vi "chirp_v0.vi"() -> ()   [LabVIEW 2014]
uses:
  <vilib>/rvi/FXPMathLib/FxpSinAndCos/XNode/nifxpmath_SinAndCos.xnode
  <vilib>/eio/EIONode/EIONode.xnode
  <vilib>/rvi/FXPMathLib/FxpMul/XNode/nifxpmath_Multiplier.xnode
  <vilib>/rvi/FXPMathLib/FxpSinAndCos/simVIs/DllFxpSinAndCosTemp_sub.vi
  <vilib>/rvi/FXPMathLib/FxpSinAndCos/subVIs/nifxpmath_SinAndCos_SimConfig.ctl
  <vilib>/rvi/eio/common/nirviEmuTemplateMethod_errors.vi
  <vilib>/rvi/FXPMathLib/sim/FxpSim.dll
  <vilib>/rvi/DataTransferAndStorage/Container/XNode/niFpgaContainer.xnode
  <vilib>/rvi/FXPMathLib/FxpSub/XNode/nifxpmath_Sub.xnode
  <vilib>/rvi/FXPMathLib/FxpAdd/XNode/nifxpmath_Add.xnode
  <vilib>/rvi/Analysis/measure/butterworth/XNode/niFpgaButterworthFilter.xnode
  <vilib>/rvi/interface/RandomDataEmulation/nirviRandomDataFpgaMultiElementTemplate.vi
panel:
  in  "Step/Chirp":bool
  in  "fb_step (N)":fxp<+/-,36,11>
  in  "initial frenqueny (Hz)":fxp<+,20,5>
  in  "target frenqueny (Hz)":fxp<+,23,8>
  in  "target time (s)":fxp<+,24,9>
  out "chirp_signal":fxp<+/-,36,11>
  out "frequency (Hz)":fxp<+,24,9>
  out "Load cell 1":fxp<+/-,60,14>
  out "Load cell 0":fxp<+/-,60,14>
  in  "xb_M_avg_Tc (uSec)":u32
  out "Omega_b(T)":fxp<+/-,20,9>
  out "Omega_b(M_avg)":fxp<+/-,32,12>
  out "Omega_b(M)":fxp<+/-,32,12>
  in  "Method case 2":i32
  out "f_LC":fxp<+/-,36,17>
  in  "Load cell reset":bool
  in  "Load cell stop":bool
  in  "Load cell start":bool
  out "fbr_d":fxp<+/-,36,13>
  in  "Sin wave amplitude (N)":fxp<+,20,11>
  out "Db_d(M_avg method)":fxp<+/-,25,10>
  in  "Db_d_M_Tc (mSec)":u32 format="%#_6f"
  out "Db_d(M method)":fxp<+/-,25,10>
  out "xb_d(M_avg method)":fxp<+/-,25,10>
  in  "Db_M_avg_Tc (uSec)":u32
  out "xb_d(M method)":fxp<+/-,25,10>
  in  "xb_d_M_Tc (mSec)":u32 format="%#_6f"
  in  "Method case":i32
  out "xb_d(T method)":fxp<+/-,25,10>
  out "Db_d(T method)":fxp<+/-,25,10>
  in  "mt0_velocity":u32
  out "mt_velocity":u32
  in  "mt0_omega":u32
  out "mt_omega":u32
  out "fbt_d":fxp<+/-,25,15>
  out "Db_d(mm/s)":fxp<+/-,25,10>
  out "Atom_Position_b":i32
  out "xb_d(mm/s)":fxp<+/-,25,10>
  in  "dF_PID_add":bool
  in  "scaled coefficients_dFb_PID":i32[](array[numeric])=[1067016412, 3362706]
  out "dFb_PID":fxp<+/-,25,15>
  out "Sin wave time (s)":fxp<+,64,32>
  in  "Atom Reset_b":bool
  out "xb(mm)":fxp<+/-,22,7>
  in  "Friction tolerance_b":fxp<+,12,4>
  in  "Coe Ini":bool
  in  "Encoder Reset_b":bool
  in  "Stop Motor_b":bool
  in  "viscous_cons_b":fxp<+/-,20,10>
  in  "fstb":fxp<+/-,15,6>
  in  "Db_d_tol":fxp<+,20,12>
  in  "Kib":fxp<+,27,10>
  in  "Kdb":fxp<+,26,2>
  in  "kb c":fxp<+,15,8>
  in  "kb t":fxp<+,15,8>
  out "fbt_i":fxp<+/-,34,18>
  in  "Kpb":fxp<+,11,7>=0.375
  in  "fv_coeff. b":fxp<+,13,1>
  out "Friction comp_b":fxp<+/-,20,10>
  in  "fcb":fxp<+/-,15,6>
  in  "fvb":fxp<+,20,12>
  out "kb":fxp<+,15,8>
  out "fb":fxp<+/-,20,10>
  out "fb_tilde":fxp<+/-,21,11>
  out "Fb_PID":fxp<+/-,21,11>
  in  "fb_tolerance":fxp<+,32,9>=1.0
  out "fbr":fxp<+/-,36,11>
  out "Encoder Position_b":i32
  out "rad(NrTheta)_b":fxp<+/-,33,18> format="%.21g"
  out "Db(mm)":fxp<+/-,22,7>
  out "Omega_b(rad/s)":fxp<+/-,20,9>
  out "vq_b_F":fxp<+/-,20,5> format="%.57g"
  out "vd_b_F":fxp<+/-,20,5>
  out "va_b":fxp<+/-,20,5> format="%.21g"
  out "vb_b":fxp<+/-,20,5> format="%.21g"
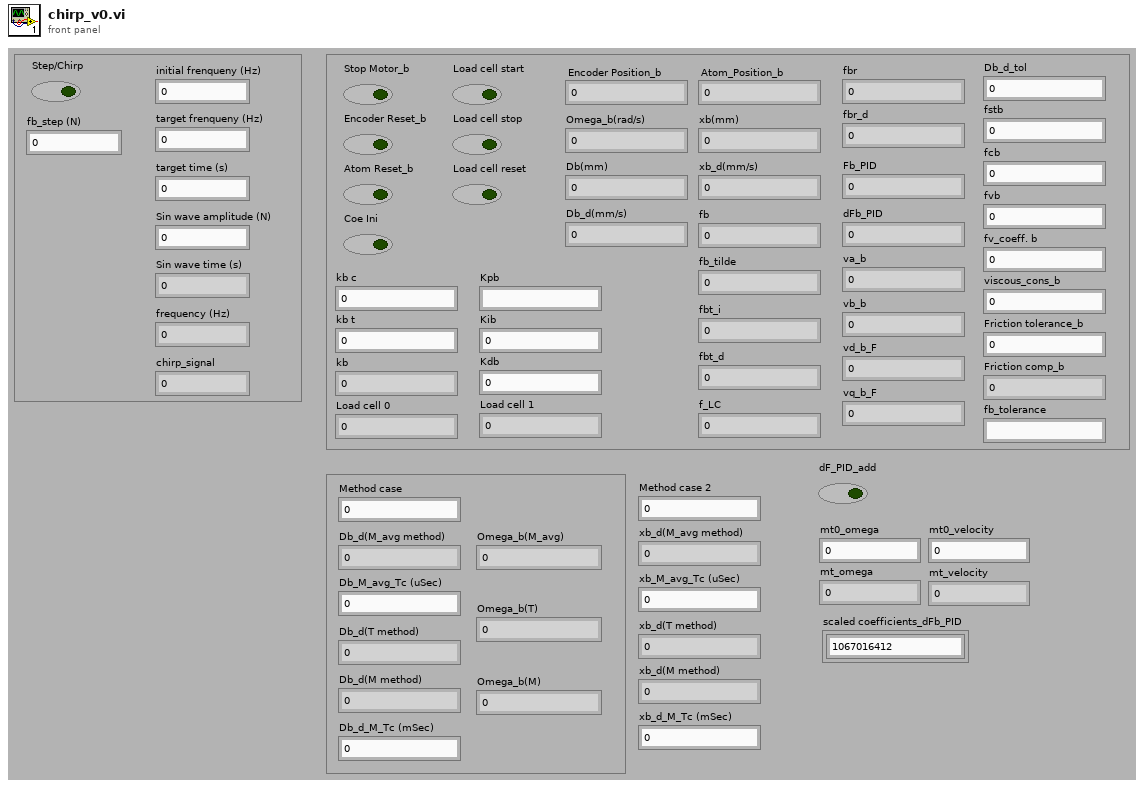
[diagram p1: front panel]
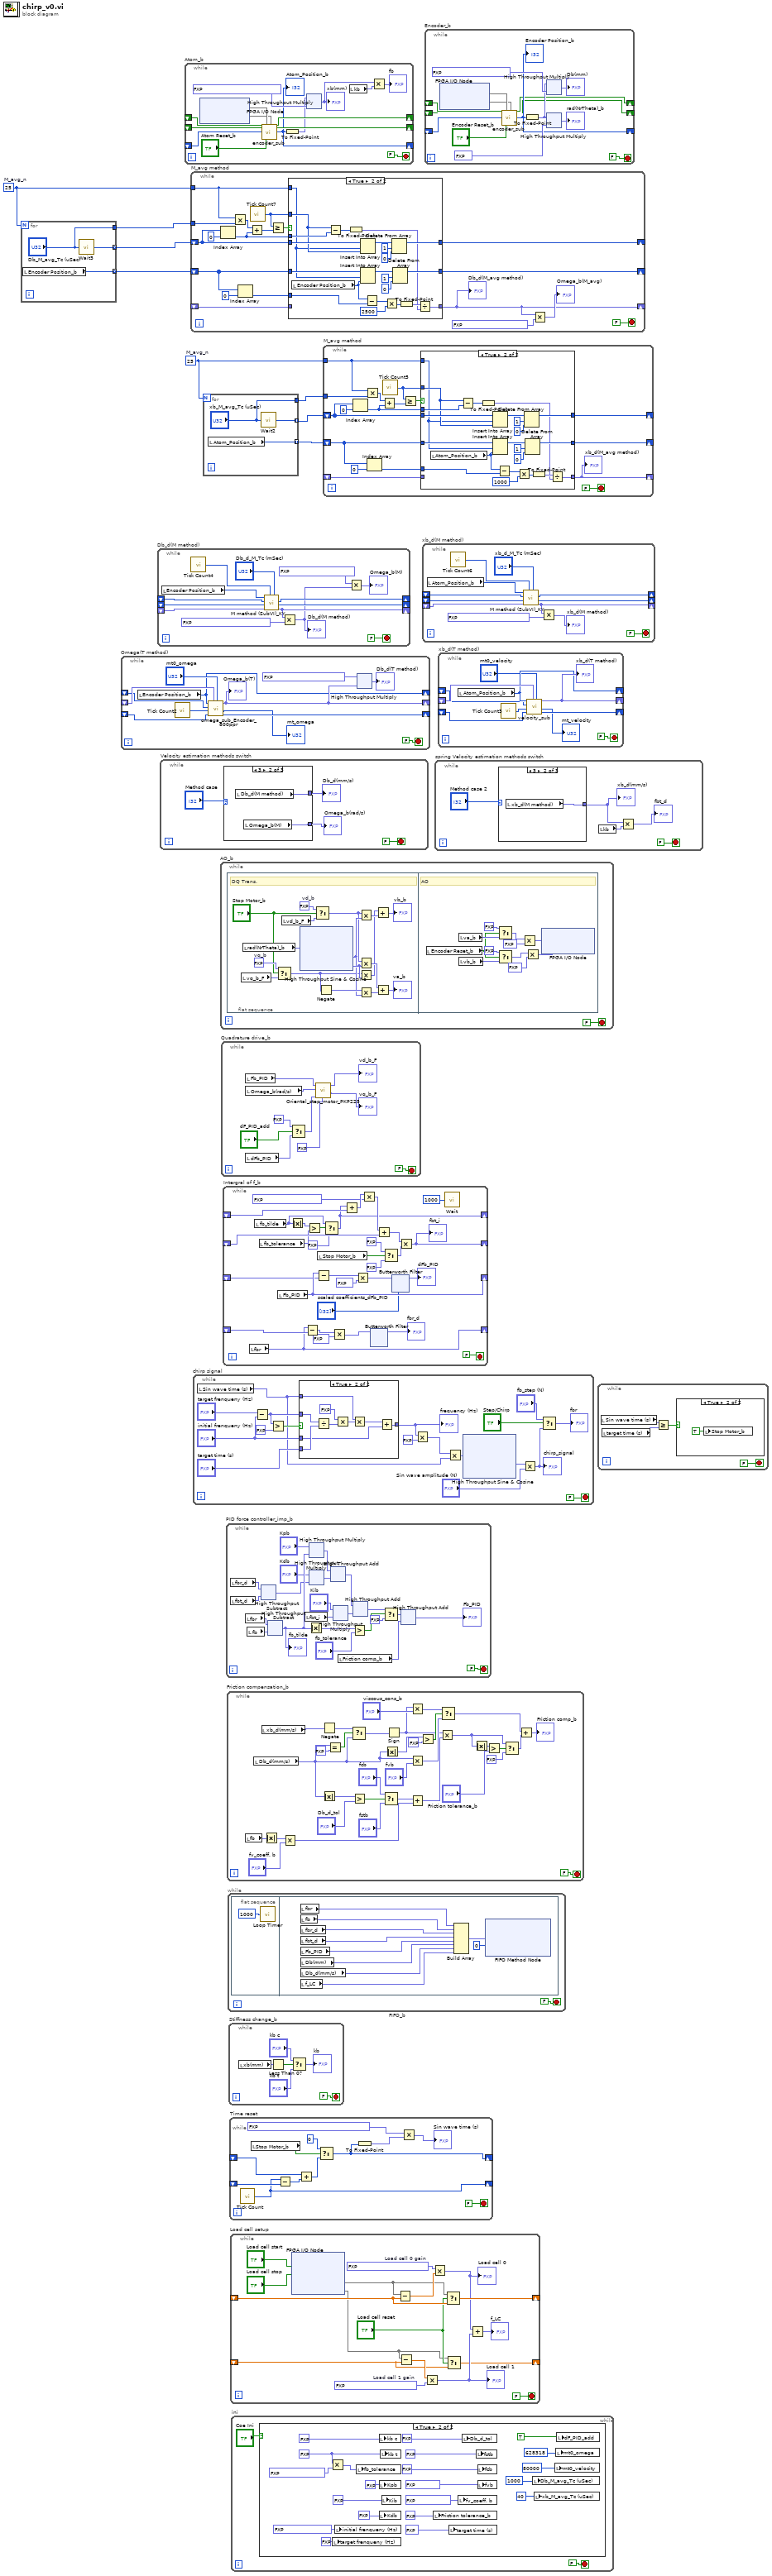
[diagram p0: block diagram]
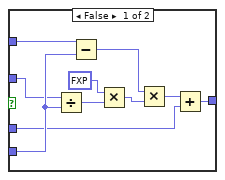
[diagram p3: hidden frame]
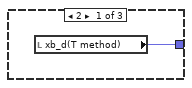
[diagram p5: hidden frame]
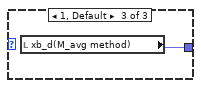
[diagram p6: hidden frame]
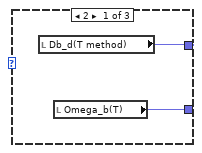
[diagram p8: hidden frame]
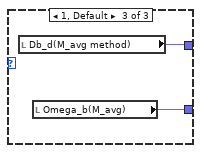
[diagram p9: hidden frame]
diagram:
  w2 = 25  # M_avg_n
  w6 = 25  # M_avg_n
  n1 = for {
    N: w6 -> [_]
    tunnel: [w11] -> w8 mode=indexing
    tunnel: [w9] -> w7 mode=indexing
    tunnel: ["Db_M_avg_Tc (uSec)"] -> w5
    n2 = local read "Encoder Position_b"() -> (w9:i32)
    n3 = call "Wait3"("Count(uSec)"="Db_M_avg_Tc (uSec)") -> ("Tick Count(uSec)"=w11:u32)
  }
  n4 = while "Omega(T method)" {
    shift-right: [w13] -> _
    shift-left: _ -> [w12]
    shift-right: [w20] -> _
    shift-left: _ -> [w14]
    shift-right: [w18] -> _
    shift-left: _ -> [w16]
    stop <- FALSE stop-if-true
    n5 = local read "Encoder Position_b"() -> (w13:i32)
    n6 = call "Tick Count2"() -> ("Tick Count(Ticks)"=w15:u32)
    n7 = call "omega_sub_Encoder_800ppr.vi"("mt0"="mt0_omega", "omega_pre"=w16, "ticks_m_pre"=w14, "ticks"=w15, "count_pre"=w12, "count"=w13) -> ("ticks_m"=w20:u32, "mt"=→"mt_omega":u32, "omega"=w18:fxp<+/-,20,9>)  [unwired: 3 in]
    "Omega_b(T)" <- w18
    n8 = xnode ("High Throughput Multiply")("x"=fxp<+/-,26,1> 0.38515496253967285, "y"=w18) -> ("x*y"=→"Db_d(T method)":fxp<+/-,24,9>)
  }
  n9 = while "Db_d(M method)" {
    shift-right: [w35] -> _
    shift-left: _ -> [w30]
    shift-right: [w34] -> _
    shift-left: _ -> [w29]
    shift-right: [w27] -> _
    shift-left: _ -> [w28]
    stop <- FALSE stop-if-true
    n10 = local read "Encoder Position_b"() -> (w31:i32)
    n11 = call "Tick Count4"() -> ("Tick Count(mSec)"=w32:u32)
    n12 = call "M method (SubVI)_KY.vi"("Tc (mSec)"="Db_d_M_Tc (mSec)", "Tick Count (mSec)"=w32, "Encoder velocity_pre (pulse/s)"=w28, "Shift Register in 2"=w29, "Shift Register in 1"=w30, "Encoder pulses"=w31) -> ("Encoder velocity (pulse/s)"=w27:fxp<+/-,64,32>, "Shift Register out 2"=w34:i32, "Shift Register out 1"=w35:u32)  [unwired: 3 in]
    n13 = Multiply(x=w27, y=fxp<+/-,20,-5> 0.002499997615814209) -> (x*y=w26:fxp<+/-,25,10>)
    "Db_d(M method)" <- w26
    n14 = Multiply(x=fxp<+/-,32,12> 3.1415929794311523, y=w26) -> (x*y=→"Omega_b(M)":fxp<+/-,32,12>)
  }
  n15 = while "Velocity estimation methods switch" {
    stop <- FALSE stop-if-true
    n16 = case shown="3" "Method case" {
      tunnel: [w42 w44 w46] -> w39
      tunnel: [w43 w45 w47] -> w38
      frame 2 {
        n17 = local read "Db_d(T method)"() -> (w42:fxp<+/-,25,10>)
        n18 = local read "Omega_b(T)"() -> (w43:fxp<+/-,20,9>)
      }
      frame 3 {
        n19 = local read "Db_d(M method)"() -> (w44:fxp<+/-,25,10>)
        n20 = local read "Omega_b(M)"() -> (w45:fxp<+/-,32,12>)
      }
      frame 1, Default {
        n21 = local read "Db_d(M_avg method)"() -> (w46:fxp<+/-,25,10>)
        n22 = local read "Omega_b(M_avg)"() -> (w47:fxp<+/-,32,12>)
      }
    }
    "Db_d(mm/s)" <- w39
    "Omega_b(rad/s)" <- w38
  }
  n23 = while "Atom_b" {
    shift-right: [w61] -> _
    shift-left: _ -> [w59]
    shift-right: [w60] -> _
    shift-left: _ -> [w58]
    shift-right: [w48] -> _
    shift-left: _ -> [w55]
    stop <- FALSE stop-if-true
    n24 = xnode "FPGA I/O Node"() -> ("Mod5/DI0"=w57, "Mod5/DI1"=w56)  [unwired: 2 in, 2 out]
    n25 = call "encoder_sub.vi"("A_pre"=w59, "B_pre"=w58, "Encoder Position_pre"=w55, "A input"=w57, "Encoder Position Reset"="Atom Reset_b", "B input"=w56) -> ("A"=w61:bool, "B"=w60:bool, "Encoder Position (Counts)"=w48:i32)  [unwired: 19 in]
    "Atom_Position_b" <- w48
    n26 = To Fixed-Point(number=w48) -> (fixed-point=w53:fxp<+/-,18,18>)  [unwired: 1 in]
    n27 = xnode ("High Throughput Multiply")("x"=w53, "y"=fxp<+/-,20,-5> 0.0009999871253967285) -> ("x*y"=w50:fxp<+/-,22,7>)
    "xb(mm)" <- w50
    n28 = local read "kb"() -> (w51:fxp<+,15,8>)
    n29 = Multiply(x=w50, y=w51) -> (x*y=→"fb":fxp<+/-,20,10>)
  }
  n30 = while "M_avg method" {
    shift-right: [w73] -> _
    shift-left: w8 -> [w76]
    tunnel: w6 -> [w74]
    shift-right: [w71] -> _
    shift-left: w7 -> [w69]
    shift-right: [w63] -> _
    shift-left: _ -> [w67]
    tunnel: w5 -> [w66]
    stop <- FALSE stop-if-true
    n31 = Index Array(array=w76, index=0) -> (element=w72:u32)
    n32 = Multiply(x=w74, y=w66) -> (x*y=w79:u32)
    n33 = Index Array(array=w69, index=0) -> (element=w68:i32)
    n34 = Add(x=w79, y=w72) -> (x+y=w78:u32)
    n35 = call "Tick Count7"() -> ("Tick Count(uSec)"=w75:u32)
    n36 = Greater Or Equal?(x=w75, y=w78) -> (x >= y?=w77:bool)
    n37 = case shown="True" w77 {
      tunnel: w76 -> [w84 w106]
      tunnel: w75 -> [_ w100]
      tunnel: w74 -> [_ w89]
      tunnel: [w84 w102] -> w73
      tunnel: w72 -> [_ w101]
      tunnel: w69 -> [w83 w90]
      tunnel: [w83 w88] -> w71
      tunnel: [w82 w87] -> w63
      tunnel: w68 -> [_ w85]
      tunnel: w67 -> [w82 _]
      frame False {
      }
      frame True {
        n38 = local read "Encoder Position_b"() -> (w94:i32)
        n39 = Subtract(x=w100, y=w101) -> (x-y=w99:u32)
        n40 = To Fixed-Point(number=w99) -> (fixed-point=w86:fxp<+,32,32>)  [unwired: 1 in]
        n41 = Insert Into Array(array=w106, index=w89, new element=w100) -> (w105:u32[])
        n42 = Insert Into Array(array=w90, index=w89, new element=w94) -> (w91:i32[])
        n43 = Subtract(x=w94, y=w85) -> (x-y=w95:i32)
        n44 = Multiply(x=w95, y=2500) -> (x*y=w97:i32)
        n45 = Delete From Array(array=w105, length=1, index=0) -> (array with subset deleted=w102:u32[])  [unwired: 1 out]
        n46 = Delete From Array(array=w91, length=1, index=0) -> (array with subset deleted=w88:i32[])  [unwired: 1 out]
        n47 = To Fixed-Point(number=w97) -> (fixed-point=w98:fxp<+/-,32,32>)  [unwired: 1 in]
        n48 = Divide(x=w98, y=w86) -> (x/y=w87:fxp<+/-,25,10>)
      }
    }
    "Db_d(M_avg method)" <- w63
    n49 = Multiply(x=w63, y=fxp<+/-,32,12> 3.1415929794311523 ("x")) -> (x*y=→"Omega_b(M_avg)":fxp<+/-,32,12>)
  }
  n50 = while "chirp signal" {
    stop <- FALSE stop-if-true
    n51 = local read "Sin wave time (s)"() -> (w107:fxp<+,64,32>)
    n52 = Subtract(x="target frenqueny (Hz)", y="initial frenqueny (Hz)") -> (x-y=w108:fxp<+/-,24,9>)
    n53 = Greater?(x=w108, y=fxp<+/-,24,9> 0.0) -> (0:w111:bool)
    n54 = case shown="True" w111 {
      tunnel: [w133 w142] -> w116
      tunnel: "target time (s)" -> [w130 w141]
      tunnel: "initial frenqueny (Hz)" -> [w129 w140]
      tunnel: w107 -> [w132 w139]
      tunnel: w108 -> [w128 w138]
      frame False {
        n55 = Divide(x=w128, y=w130) -> (x/y=w127:fxp<+/-,24,9>)
        n56 = Subtract(x=w132, y=w130) -> (x-y=w131:fxp<+/-,24,9>)
        n57 = Multiply(x=fxp<+/-,24,9> 0.5, y=w127) -> (x*y=w126:fxp<+/-,23,10>)
        n58 = Multiply(x=w131, y=w126) -> (x*y=w134:fxp<+/-,26,11>)
        n59 = Add(x=w134, y=w129) -> (x+y=w133:fxp<+,24,9>)
      }
      frame True {
        n60 = Divide(x=w138, y=w141) -> (x/y=w136:fxp<+/-,24,9>)
        n61 = Multiply(x=fxp<+/-,24,9> 0.5, y=w136) -> (x*y=w137:fxp<+/-,23,10>)
        n62 = Multiply(x=w139, y=w137) -> (x*y=w143:fxp<+/-,26,11>)
        n63 = Add(x=w143, y=w140) -> (x+y=w142:fxp<+,24,9>)
      }
    }
    "frequency (Hz)" <- w116
    n64 = Multiply(x=w116, y=fxp<+,1,2> 2.0) -> (x*y=w123:fxp<+,25,10>)
    n65 = Multiply(x=w123, y=w107) -> (x*y=w115:fxp<+,33,18>)
    n66 = xnode "High Throughput Sine & Cosine"("x (pi)"=w115) -> ("sin(x)"=w114:fxp<+/-,16,2>)  [unwired: 1 out]
    n67 = Multiply(x=w114, y="Sin wave amplitude (N)") -> (x*y=w119:fxp<+/-,36,11>)
    "chirp_signal" <- w119
    n68 = Select(t="fb_step (N)", s="Step/Chirp", f=w119) -> (s? t:f=→"fbr":fxp<+/-,36,11>)
  }
  n69 = for {
    N: w2 -> [_]
    tunnel: [w176] -> w1 mode=indexing
    tunnel: ["xb_M_avg_Tc (uSec)"] -> w3
    tunnel: [w174] -> w4 mode=indexing
    n70 = local read "Atom_Position_b"() -> (w174:i32)
    n71 = call "Wait2"("Count(uSec)"="xb_M_avg_Tc (uSec)") -> ("Tick Count(uSec)"=w176:u32)
  }
  n72 = while "AO_b" {
    stop <- FALSE stop-if-true
    n73 = flat-sequence {
      frame #0 {
        w184 = fxp<+/-,20,5> 0.0  # vq_b
        w183 = fxp<+/-,20,5> 0.0  # vd_b
        # "DQ Trans."
        n74 = local read "vq_b_F"() -> (w181:fxp<+/-,20,5>)
        n75 = local read "rad(NrTheta)_b"() -> (w194:fxp<+/-,33,18>)
        n76 = Select(t=w184, s="Stop Motor_b", f=w181) -> (s? t:f=w178:fxp<+/-,20,5>)
        n77 = local read "vd_b_F"() -> (w182:fxp<+/-,20,5>)
        n78 = xnode "High Throughput Sine & Cosine"("x (pi)"=w194) -> ("sin(x)"=w185:fxp<+/-,17,2>, "cos(x)"=w186:fxp<+/-,17,2>)
        n79 = Select(t=w183, s="Stop Motor_b", f=w182) -> (s? t:f=w179:fxp<+/-,20,5>)
        n80 = Negate(x=w178) -> (-x=w193:fxp<+/-,21,6>)
        n81 = Multiply(x=w179, y=w185) -> (x*y=w189:fxp<+/-,20,5>)
        n82 = Multiply(x=w179, y=w186) -> (x*y=w192:fxp<+/-,20,5>)
        n83 = Multiply(x=w178, y=w186) -> (x*y=w188:fxp<+/-,20,5>)
        n84 = Multiply(x=w193, y=w185) -> (x*y=w191:fxp<+/-,20,5>)
        n85 = Add(x=w188, y=w189) -> (x+y=→"vb_b":fxp<+/-,20,5>)
        n86 = Add(x=w192, y=w191) -> (x+y=→"va_b":fxp<+/-,20,5>)
      }
      frame #1 {
        # "AO"
        n87 = local read "Encoder Reset_b"() -> (w231:bool)
        n88 = local read "va_b"() -> (w232:fxp<+/-,20,5>)
        n89 = local read "vb_b"() -> (w233:fxp<+/-,20,5>)
        n90 = Select(t=fxp<+/-,20,5> 3.0 ("Mod2/AO4"), s=w231, f=w232) -> (s? t:f=w229:fxp<+/-,20,5>)
        n91 = Select(t=fxp<+/-,20,5> 0.0 ("Mod2/AO4"), s=w231, f=w233) -> (s? t:f=w226:fxp<+/-,20,5>)
        n92 = Multiply(x=w229, y=fxp<+/-,20,5> -0.5) -> (x*y=w230:fxp<+/-,20,5>)
        n93 = Multiply(x=w226, y=fxp<+/-,20,5> -0.5) -> (x*y=w225:fxp<+/-,20,5>)
        n94 = xnode "FPGA I/O Node"("Mod2/AO0"=w230, "Mod2/AO1"=w225) -> ()  [unwired: 2 in, 2 out]
      }
    }
  }
  n95 = while "Quadrature drive_b" {
    stop <- FALSE stop-if-true
    n96 = local read "Fb_PID"() -> (w239:fxp<+/-,21,11>)
    n97 = local read "Omega_b(rad/s)"() -> (w238:fxp<+/-,20,9>)
    n98 = local read "dFb_PID"() -> (w242:fxp<+/-,25,15>)
    n99 = Select(t=fxp<+/-,25,15> 0.0 ("f"), s="dF_PID_add", f=w242) -> (s? t:f=w237:fxp<+/-,25,15>)
    n100 = call "Oriental_step_motor_PKP225.vi"("F_Threshold"=fxp<+,12,12> 10.0, "dFmr"=w237, "omega"=w238, "Fmr"=w239) -> ("vq_F"=→"vq_b_F":fxp<+/-,20,5>, "vd_F"=→"vd_b_F":fxp<+/-,20,5>)  [unwired: 6 in]
  }
  n101 = while "Intergral of f_b" {
    shift-right: [w265] -> _
    shift-left: _ -> [w266]
    shift-right: [w247] -> _
    shift-left: _ -> [w271]
    shift-right: [w261] -> _
    shift-left: _ -> [w259]
    shift-right: [w251] -> _
    shift-left: _ -> [w252]
    stop <- FALSE stop-if-true
    n102 = local read "fbr"() -> (w251:fxp<+/-,36,11>)
    n103 = local read "fb_tilde"() -> (w267:fxp<+/-,21,11>)
    n104 = local read "fb_tolerance"() -> (w269:fxp<+,32,9>)
    n105 = local read "Fb_PID"() -> (w261:fxp<+/-,21,11>)
    n106 = Absolute Value(x=w267) -> (abs(x)=w270:fxp<+,21,11>)
    n107 = Subtract(x=w251, y=w252) -> (x-y=w254:fxp<+/-,37,12>)
    n108 = Greater?(x=w270, y=w269) -> (0:w268:bool)
    n109 = Subtract(x=w261, y=w259) -> (x-y=w260:fxp<+/-,22,12>)
    n110 = local read "Stop Motor_b"() -> (w273:bool)
    n111 = Select(t=w267, s=w268, f=fxp<+/-,21,11> 0.0) -> (s? t:f=w265:fxp<+/-,21,11>)
    n112 = Multiply(x=w254, y=fxp<+/-,24,11> 1000.0) -> (x*y=w253:fxp<+/-,25,15>)
    n113 = Add(x=w265, y=w266) -> (x+y=w275:fxp<+/-,22,12>)
    n114 = Multiply(x=w260, y=fxp<+,10,10> 1000.0) -> (x*y=w258:fxp<+/-,25,15>)
    n115 = Multiply(x=w275, y=fxp<+/-,30,12> 0.000499725341796875) -> (x*y=w272:fxp<+/-,25,15>)
    n116 = xnode "Butterworth Filter"("input data"=w253) -> ("output data"=→"fbr_d":fxp<+/-,25,15>)  [unwired: 2 in]
    n117 = Add(x=w272, y=w271) -> (x+y=w248:fxp<+/-,32,16>)
    n118 = Select(t=fxp<+/-,2,2> 0.0, s=w273, f=fxp<+/-,2,2> 1.0) -> (s? t:f=w249:fxp<+/-,2,2>)
    n119 = xnode "Butterworth Filter"("input data"=w258, "scaled coefficients"="scaled coefficients_dFb_PID") -> ("output data"=→"dFb_PID":fxp<+/-,25,15>)  [unwired: 1 in]
    n120 = Multiply(x=w248, y=w249) -> (x*y=w247:fxp<+/-,34,18>)
    "fbt_i" <- w247
    n121 = call "Wait"("Count(uSec)"=u32 1000 ("Count(mSec)")) -> ()  [unwired: 1 out]
  }
  n122 = while "PID force controller_imp_b" {
    stop <- FALSE stop-if-true
    n123 = local read "fbr_d"() -> (w294:fxp<+/-,36,13>)
    n124 = local read "fbt_d"() -> (w295:fxp<+/-,25,15>)
    n125 = local read "fbr"() -> (w298:fxp<+/-,36,11>)
    n126 = local read "fb"() -> (w309:fxp<+/-,20,10>)
    n127 = xnode "High Throughput Subtract"("x"=w294, "y"=w295) -> ("x-y"=w296:fxp<+/-,39,16>)
    n128 = xnode "High Throughput Subtract"("x"=w298, "y"=w309) -> ("x-y"=w311:fxp<+/-,37,12>)
    "fb_tilde" <- w311
    n129 = local read "fbt_i"() -> (w307:fxp<+/-,34,18>)
    n130 = Absolute Value(x=w311) -> (abs(x)=w314:fxp<+,37,12>)
    n131 = xnode ("High Throughput Multiply")("x"="Kpb", "y"=w311) -> ("x*y"=w310:fxp<+/-,33,17>)
    n132 = xnode ("High Throughput Multiply")("x"="Kdb", "y"=w296) -> ("x*y"=w304:fxp<+/-,31,21>)
    n133 = xnode ("High Throughput Add")("x"=w310, "y"=w304) -> ("x+y"=w308:fxp<+/-,21,11>)
    n134 = xnode ("High Throughput Multiply")("x"="Kib", "y"=w307) -> ("x*y"=w306:fxp<+/-,31,14>)
    n135 = local read "Friction comp_b"() -> (w302:fxp<+/-,20,10>)
    n136 = Greater?(x=w314, y="fb_tolerance") -> (0:w313:bool)
    n137 = xnode ("High Throughput Add")("x"=w308, "y"=w306) -> ("x+y"=w305:fxp<+/-,21,11>)
    n138 = Select(t=w305, s=w313, f=fxp<+/-,20,10> 0.0) -> (s? t:f=w303:fxp<+/-,21,11>)
    n139 = xnode ("High Throughput Add")("x"=w303, "y"=w302) -> ("x+y"=→"Fb_PID":fxp<+/-,21,11>)
  }
  n140 = while "Friction compensation_b" {
    stop <- FALSE stop-if-true
    n141 = local read "fb"() -> (w346:fxp<+/-,20,10>)
    n142 = local read "Db_d(mm/s)"() -> (w327:fxp<+/-,25,10>)
    n143 = local read "xb_d(mm/s)"() -> (w324:fxp<+/-,25,10>)
    n144 = Absolute Value(x=w346) -> (abs(x)=w347:fxp<+,20,10>)
    n145 = Multiply(x=w347, y="fv_coeff. b") -> (x*y=w344:fxp<+/-,20,10>)
    n146 = Negate(x=w324) -> (-x=w323:fxp<+/-,26,11>)
    n147 = Absolute Value(x=w327) -> (abs(x)=w341:fxp<+,25,10>)
    n148 = Equal?(x=w327, y=fxp<+/-,25,15> 0.0) -> (x = y?=w328:bool)
    n149 = Select(t=w323, s=w328, f=w327) -> (s? t:f=w326:fxp<+/-,26,11>)
    n150 = Greater?(x=w341, y="Db_d_tol") -> (0:w340:bool)
    n151 = Select(t="fcb", s=w340, f="fstb") -> (s? t:f=w338:fxp<+/-,15,6>)
    n152 = Absolute Value(x=w327) -> (abs(x)=w335:fxp<+,25,10>)
    n153 = Sign(1:w326) -> (0:w325:fxp<+/-,2,2>)
    n154 = Multiply(x=w325, y="viscous_cons_b") -> (x*y=w330:fxp<+/-,20,10>)
    n155 = Multiply(x=w327, y="fvb") -> (x*y=w333:fxp<+/-,20,10>)
    n156 = Add(x=w338, y=w344) -> (x+y=w343:fxp<+/-,20,10>)
    n157 = Greater?(x=w335, y=fxp<+/-,25,15> 25.0) -> (0:w334:bool)
    n158 = Multiply(x=w325, y=w343) -> (x*y=w319:fxp<+/-,20,10>)
    n159 = Select(t=w330, s=w334, f=w333) -> (s? t:f=w332:fxp<+/-,20,10>)
    n160 = Absolute Value(x=w319) -> (abs(x)=w321:fxp<+,20,10>)
    n161 = Greater?(x=w321, y="Friction tolerance_b") -> (0:w322:bool)
    n162 = Select(t=w319, s=w322, f=fxp<+/-,20,10> 0.0) -> (s? t:f=w318:fxp<+/-,20,10>)
    n163 = Add(x=w332, y=w318) -> (x+y=→"Friction comp_b":fxp<+/-,20,10>)
  }
  n164 = while "FIFO_b" {
    stop <- FALSE stop-if-true
    n165 = flat-sequence {
      frame #0 {
        n166 = call "Loop Timer"("Count(uSec)"=u32 1000 ("Loop Period (usec)")) -> ()  [unwired: 1 out]
      }
      frame #1 {
        n167 = local read "fbr"() -> (w358:fxp<+/-,36,11>)
        n168 = local read "fb"() -> (w357:fxp<+/-,20,10>)
        n169 = local read "fbr_d"() -> (w356:fxp<+/-,36,13>)
        n170 = local read "fbt_d"() -> (w362:fxp<+/-,25,15>)
        n171 = local read "Fb_PID"() -> (w355:fxp<+/-,21,11>)
        n172 = local read "Db(mm)"() -> (w353:fxp<+/-,22,7>)
        n173 = local read "Db_d(mm/s)"() -> (w354:fxp<+/-,25,10>)
        n174 = local read "f_LC"() -> (w361:fxp<+/-,36,17>)
        n175 = Build Array(w358, w357, w356, w362, w355, w353, w354, w361) -> (w359:fxp<+/-,42,17>[])
        n176 = xnode ("FIFO Method Node")("Element"=w359, "Timeout"=0) -> ()  [unwired: 1 in, 2 out]
      }
    }
  }
  n177 = while "Stiffness change_b" {
    stop <- FALSE stop-if-true
    n178 = local read "xb(mm)"() -> (w368:fxp<+/-,22,7>)
    n179 = Less Than 0?(x=w368) -> (x < 0?=w367:bool)
    n180 = Select(t="kb c", s=w367, f="kb t") -> (s? t:f=→"kb":fxp<+,15,8>)
  }
  n181 = while "Time reset" {
    shift-right: [w379] -> _
    shift-left: _ -> [w380]
    shift-right: [w371] -> _
    shift-left: _ -> [w373]
    stop <- FALSE stop-if-true
    n182 = call "Tick Count"() -> ("Tick Count(uSec)"=w379:u32)
    n183 = local read "Stop Motor_b"() -> (w376:bool)
    n184 = Subtract(x=w379, y=w380) -> (x-y=w375:u32)
    n185 = Add(x=w373, y=w375) -> (x+y=w374:u32)
    n186 = Select(t=u32 0, s=w376, f=w374) -> (s? t:f=w371:u32)
    n187 = To Fixed-Point(number=w371) -> (fixed-point=w369:fxp<+,64,32>)  [unwired: 1 in]
    n188 = Multiply(x=fxp<+,20,-18> 1.0000003385357559e-06 ("y"), y=w369) -> (x*y=→"Sin wave time (s)":fxp<+,64,32>)
  }
  n189 = while "Load cell setup" {
    shift-right: [w394] -> _
    shift-left: _ -> [w391]
    shift-right: [w388] -> _
    shift-left: _ -> [w384]
    stop <- FALSE stop-if-true
    w382 = fxp<+/-,36,18> 48771.92979812622  # Load cell 0 gain
    w381 = fxp<+/-,36,18> 47087.49039840698  # Load cell 1 gain
    n190 = xnode "FPGA I/O Node"("Mod4/Start"="Load cell start", "Mod4/Stop"="Load cell stop") -> ("Mod4/AI0"=w392, "Mod4/AI1"=w385)  [unwired: 4 in, 4 out]
    n191 = Subtract(x=w392, y=w391) -> (x-y=w393:dbl)
    n192 = Subtract(x=w385, y=w384) -> (x-y=w386:dbl)
    n193 = Multiply(x=w386, y=w381) -> (x*y=w389:fxp<+/-,64,36>)
    "Load cell 1" <- w389
    n194 = Multiply(x=w382, y=w393) -> (x*y=w390:fxp<+/-,64,36>)
    "Load cell 0" <- w390
    n195 = Select(t=w392, s="Load cell reset", f=w391) -> (s? t:f=w394:dbl)
    n196 = Select(t=w385, s="Load cell reset", f=w384) -> (s? t:f=w388:dbl)
    n197 = Add(x=w390, y=w389) -> (x+y=→"f_LC":fxp<+/-,36,17>)
  }
  n198 = while "ini" {
    stop <- FALSE stop-if-true
    n199 = case shown="True" "Coe Ini" {
      frame False {
      }
      frame True {
        w411 = fxp<+,15,8> 58.0 ("kb")
        n200 = Multiply(x=w411, y=fxp<+,17,1> 0.00250244140625 ("kb")) -> (x*y=w412:fxp<+,32,9>)
        n201 = local write "target frenqueny (Hz)"(fxp<+,23,8> 10.0 ("target frenqueny (Hz)")) -> ()
        n202 = local write "initial frenqueny (Hz)"(fxp<+,20,5> 0.100006103515625 ("initial frenqueny (Hz)")) -> ()
        n203 = local write "fb_tolerance"(w412) -> ()
        n204 = local write "kb c"(fxp<+,15,8> 58.0 ("kb")) -> ()
        n205 = local write "Kpb"(fxp<+,11,7> 80.0 ("Kpb")) -> ()
        n206 = local write "Kdb"(fxp<+,26,2> 0.5 ("Kdy 2")) -> ()
        n207 = local write "kb t"(w411) -> ()
        n208 = local write "Kib"(fxp<+,27,10> 40.0 ("Kiy 2")) -> ()
        n209 = local write "Friction tolerance_b"(fxp<+,12,4> 10.0 ("Friction tolerance_y")) -> ()
        n210 = local write "target time (s)"(fxp<+,24,9> 120.0 ("target time (s)")) -> ()
        n211 = local write "fv_coeff. b"(fxp<+,13,1> 0.14990234375 ("fv_coeff. y")) -> ()
        n212 = local write "Db_d_tol"(fxp<+,20,12> 1.0 ("Dy_d_tol")) -> ()
        n213 = local write "fstb"(fxp<+/-,15,6> 12.0 ("fsty")) -> ()
        n214 = local write "fcb"(fxp<+/-,15,6> 8.0 ("fcy")) -> ()
        n215 = local write "fvb"(fxp<+,20,12> 0.19921875 ("fvy")) -> ()
        n216 = local write "Db_M_avg_Tc (uSec)"(u32 1000 ("M_avg_Tc (uSec)")) -> ()
        n217 = local write "xb_M_avg_Tc (uSec)"(u32 40 ("M_avg_Tc (uSec)")) -> ()
        n218 = local write "mt0_velocity"(u32 80000 ("mt0_velocity")) -> ()
        n219 = local write "mt0_omega"(u32 628318 ("mt0_omega")) -> ()
        n220 = local write "dF_PID_add"(TRUE ("dF_PID_add")) -> ()
      }
    }
  }
  n221 = while "M_avg method" {
    shift-right: [w428] -> _
    shift-left: w1 -> [w431]
    shift-right: [w423] -> _
    shift-left: w4 -> [w425]
    tunnel: w2 -> [w429]
    shift-right: [w421] -> _
    shift-left: _ -> [w424]
    tunnel: w3 -> [w422]
    stop <- FALSE stop-if-true
    n222 = Index Array(array=w431, index=0) -> (element=w427:u32)
    n223 = Multiply(x=w429, y=w422) -> (x*y=w434:u32)
    n224 = Index Array(array=w425, index=0) -> (element=w426:i32)
    n225 = Add(x=w434, y=w427) -> (x+y=w433:u32)
    n226 = call "Tick Count5"() -> ("Tick Count(uSec)"=w430:u32)
    n227 = Greater Or Equal?(x=w430, y=w433) -> (x >= y?=w432:bool)
    n228 = case shown="True" w432 {
      tunnel: w431 -> [w440 w462]
      tunnel: w430 -> [_ w456]
      tunnel: w429 -> [_ w442]
      tunnel: [w440 w458] -> w428
      tunnel: w427 -> [_ w457]
      tunnel: w425 -> [w439 w453]
      tunnel: w426 -> [_ w449]
      tunnel: [w438 w444] -> w421
      tunnel: w424 -> [w438 _]
      tunnel: [w439 w443] -> w423
      frame False {
      }
      frame True {
        n229 = local read "Atom_Position_b"() -> (w450:i32)
        n230 = Subtract(x=w456, y=w457) -> (x-y=w455:u32)
        n231 = To Fixed-Point(number=w455) -> (fixed-point=w441:fxp<+,32,32>)  [unwired: 1 in]
        n232 = Insert Into Array(array=w462, index=w442, new element=w456) -> (w461:u32[])
        n233 = Insert Into Array(array=w453, index=w442, new element=w450) -> (w454:i32[])
        n234 = Subtract(x=w450, y=w449) -> (x-y=w448:i32)
        n235 = Multiply(x=w448, y=1000) -> (x*y=w446:i32)
        n236 = Delete From Array(array=w461, length=1, index=0) -> (array with subset deleted=w458:u32[])  [unwired: 1 out]
        n237 = Delete From Array(array=w454, length=1, index=0) -> (array with subset deleted=w443:i32[])  [unwired: 1 out]
        n238 = To Fixed-Point(number=w446) -> (fixed-point=w445:fxp<+/-,32,32>)  [unwired: 1 in]
        n239 = Divide(x=w445, y=w441) -> (x/y=w444:fxp<+/-,25,10>)
      }
    }
    "xb_d(M_avg method)" <- w421
  }
  n240 = while "xb_d(M method)" {
    shift-right: [w471] -> _
    shift-left: _ -> [w466]
    shift-right: [w470] -> _
    shift-left: _ -> [w465]
    shift-right: [w463] -> _
    shift-left: _ -> [w464]
    stop <- FALSE stop-if-true
    n241 = local read "Atom_Position_b"() -> (w467:i32)
    n242 = call "Tick Count6"() -> ("Tick Count(mSec)"=w468:u32)
    n243 = call "M method (SubVI)_KY.vi"("Tc (mSec)"="xb_d_M_Tc (mSec)", "Tick Count (mSec)"=w468, "Encoder velocity_pre (pulse/s)"=w464, "Shift Register in 2"=w465, "Shift Register in 1"=w466, "Encoder pulses"=w467) -> ("Encoder velocity (pulse/s)"=w463:fxp<+/-,64,32>, "Shift Register out 2"=w470:i32, "Shift Register out 1"=w471:u32)  [unwired: 3 in]
    n244 = Multiply(x=w463, y=fxp<+/-,20,-5> 0.009999990463256836) -> (x*y=→"xb_d(M method)":fxp<+/-,25,10>)
  }
  n245 = while "Encoder_b" {
    shift-right: [w476] -> _
    shift-left: _ -> [w488]
    shift-right: [w475] -> _
    shift-left: _ -> [w487]
    shift-right: [w480] -> _
    shift-left: _ -> [w486]
    stop <- FALSE stop-if-true
    n246 = xnode "FPGA I/O Node"() -> ("Mod5/DI3"=w478, "Mod5/DI4"=w477)  [unwired: 2 in, 2 out]
    n247 = call "encoder_sub.vi"("A_pre"=w488, "B_pre"=w487, "Encoder Position_pre"=w486, "A input"=w478, "Encoder Position Reset"="Encoder Reset_b", "B input"=w477) -> ("A"=w476:bool, "B"=w475:bool, "Encoder Position (Counts)"=w480:i32)  [unwired: 19 in]
    "Encoder Position_b" <- w480
    n248 = To Fixed-Point(number=w480) -> (fixed-point=w483:fxp<+/-,18,18>)  [unwired: 1 in]
    n249 = xnode ("High Throughput Multiply")("x"=w483, "y"=fxp<+/-,15,-7> 0.0025000572204589844) -> ("x*y"=→"Db(mm)":fxp<+/-,22,7>)
    n250 = xnode ("High Throughput Multiply")("x"=w483, "y"=fxp<+,24,0> 0.125) -> ("x*y"=→"rad(NrTheta)_b":fxp<+/-,33,18>)
  }
  n251 = while "spring Velocity estimation methods switch" {
    stop <- FALSE stop-if-true
    n252 = case shown="3" "Method case 2" {
      tunnel: [w495 w496 w497] -> w491
      frame 2 {
        n253 = local read "xb_d(T method)"() -> (w495:fxp<+/-,25,10>)
      }
      frame 3 {
        n254 = local read "xb_d(M method)"() -> (w496:fxp<+/-,25,10>)
      }
      frame 1, Default {
        n255 = local read "xb_d(M_avg method)"() -> (w497:fxp<+/-,25,10>)
      }
    }
    "xb_d(mm/s)" <- w491
    n256 = local read "kb"() -> (w490:fxp<+,15,8>)
    n257 = Multiply(x=w491, y=w490) -> (x*y=→"fbt_d":fxp<+/-,25,15>)
  }
  n258 = while "xb_d(T method)" {
    shift-right: [w503] -> _
    shift-left: _ -> [w502]
    shift-right: [w505] -> _
    shift-left: _ -> [w500]
    shift-right: [w506] -> _
    shift-left: _ -> [w504]
    stop <- FALSE stop-if-true
    n259 = local read "Atom_Position_b"() -> (w503:i32)
    n260 = call "Tick Count3"() -> ("Tick Count(Ticks)"=w501:u32)
    n261 = call "velocity_sub.vi"("mt0"="mt0_velocity", "velocity_pre"=w504, "ticks_m_pre"=w500, "ticks"=w501, "count_pre"=w502, "count"=w503) -> ("ticks_m"=w505:u32, "mt"=→"mt_velocity":u32, "velocity (mm/s)"=w506:fxp<+/-,25,10>)  [unwired: 3 in]
    "xb_d(T method)" <- w506
  }
  n262 = while {
    stop <- FALSE stop-if-true
    n263 = local read "Sin wave time (s)"() -> (w510:fxp<+,64,32>)
    n264 = local read "target time (s)"() -> (w509:fxp<+,24,9>)
    n265 = Greater Or Equal?(x=w510, y=w509) -> (x >= y?=w508:bool)
    n266 = case shown="True" w508 {
      frame False {
      }
      frame True {
        n267 = local write "Stop Motor_b"(TRUE ("Stop Motor_b")) -> ()
      }
    }
  }
